vi "Get Demo Mode.vi"() -> (3 "Demo Mode":bool)   [LabVIEW 2014, in "hhVI.lvlib"]
doc: "Returns if the robot needs to have less power for use at demos."
uses:
  <vilib>/Rock Robotics/Network Tables/SD Read Boolean.vi
  hhVI.lvlib
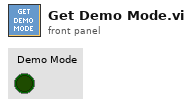
[diagram p1: front panel]
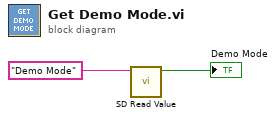
[diagram p0: block diagram]
diagram:
  n1 = call-poly <vilib>:"SD Read Value.vi"("Name"="Demo Mode") -> ("Boolean"=→"Demo Mode":bool)  [unwired: 8 in, 2 out]
